vi "Call Matlab Function.vi"(8 "error in (no error)":errorcluster, 9 "Matlab Param Array":cluster{"Name":string, "Data":variant}[](array[cluster]), 10 "Function name":string="netStartTrial", 11 "TrialBasedExperiment in":refnum<class "TrialBasedExperiment.lvclass">) -> (0 "error out":errorcluster, 1 "Return value struct":cluster{"Name":string, "Data":variant}[](array[cluster]), 2 "Return value I32":i32, 3 "TrialBasedExperiment out":refnum<class "TrialBasedExperiment.lvclass">)   [LabVIEW 2010, in "TrialBasedExperiment.lvclass"]
uses:
  TrialBasedExperiment.lvclass
  Matlab API/Matlab API.lvlib
  Core SubVIs/Core SubVIs.lvlib
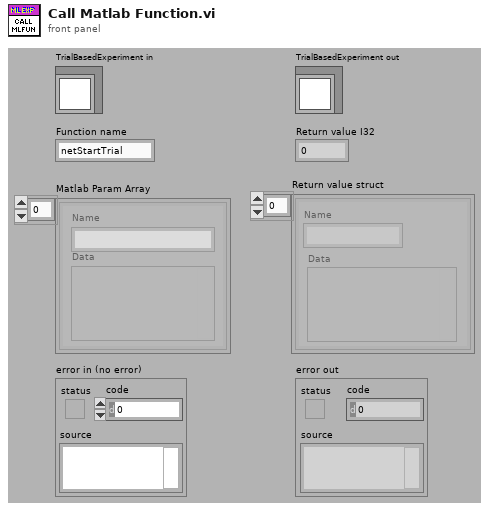
[diagram p1: front panel]
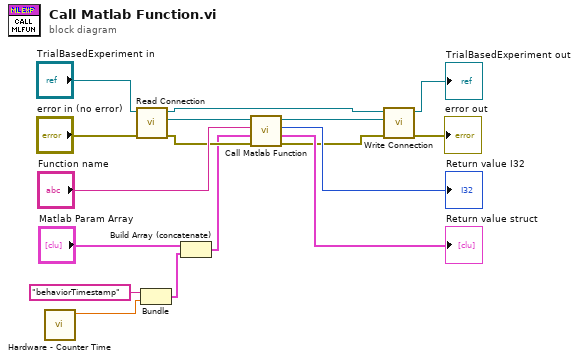
[diagram p0: block diagram]
diagram:
  n1 = call "Hardware - Counter Time.vi"() -> ("Timer Value (ms)"=w5:dbl)  [unwired: 3 in, 8 out]
  n2 = call-dynamic "Read Connection.vi"("error in (no error)"="error in (no error)", "TrialBasedExperiment in"="TrialBasedExperiment in") -> ("error out"=w12:errorcluster, "Connection"=w14:refnum<k5>, "TrialBasedExperiment out"=w17:refnum<class "TrialBasedExperiment.lvclass">)  [unwired: 7 in]
  n3 = Bundle("behaviorTimestamp", "Timer Value (ms)"=w5) -> (w3:cluster{string, "Timer Value (ms)":dbl})  [unwired: 1 out]
  n4 = Build Array (concatenate)("Matlab Param Array", w3) -> (w1:cluster{"Name":string, "Data":variant}[])
  n5 = call "Call Matlab Function.vi"("error in (no error)"=w12, "Matlab Param Array"=w1, "Function name"="Function name", "TCP Network Connection Refnum"=w14) -> ("error out"=w6:errorcluster, "Return value struct"=→"Return value struct":cluster{"Name":string, "Data":variant}[], "Return value I32"=→"Return value I32":i32, "connection ID out"=w7:refnum<k5>)  [unwired: 4 out]
  n6 = call-dynamic "Write Connection.vi"("error in (no error)"=w6, "Connection"=w7, "TrialBasedExperiment in"=w17) -> ("error out"=→"error out":errorcluster, "TrialBasedExperiment out"=→"TrialBasedExperiment out":refnum<class "TrialBasedExperiment.lvclass">)  [unwired: 7 in]
